vi "LvMPDC_SUB_SettingDialog.vi"(9 "Setting":T1) -> (1 "Setting out":T1, 2 "Caccel?":bool)   [LabVIEW 2012]
uses:
  LvMPDC_Typdef_Setting.ctl
  <vilib>/Utility/miscctls.llb/LVPointTypeDef.ctl
panel:
  in  "btn Test":bool
  in  "btn Cancel":bool
  in  "btn OK":bool
  in  "Port":u16=6600 caption="Port:"
  in  "server":string caption="Address:"
  # "MPD Server"
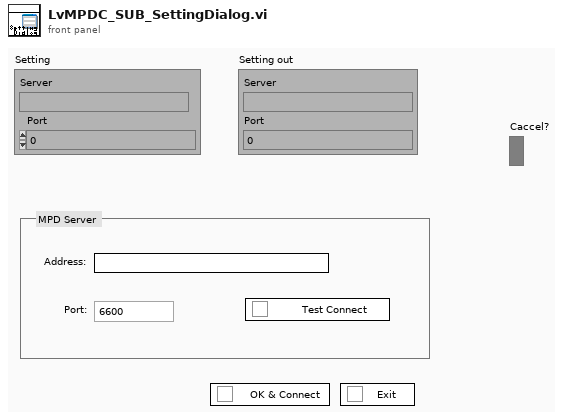
[diagram p1: front panel]
types:
  T1 = typedef "LvMPDC_Typdef_Setting.ctl" = cluster{"Server":string, "Port":u16}
  T2 = typedef "LVPointTypeDef.ctl" = cluster{"Horizontal":i16, "Vertical":i16}
  T3 = enum8{"Enabled", "Disabled", "Disabled and Grayed Out"}
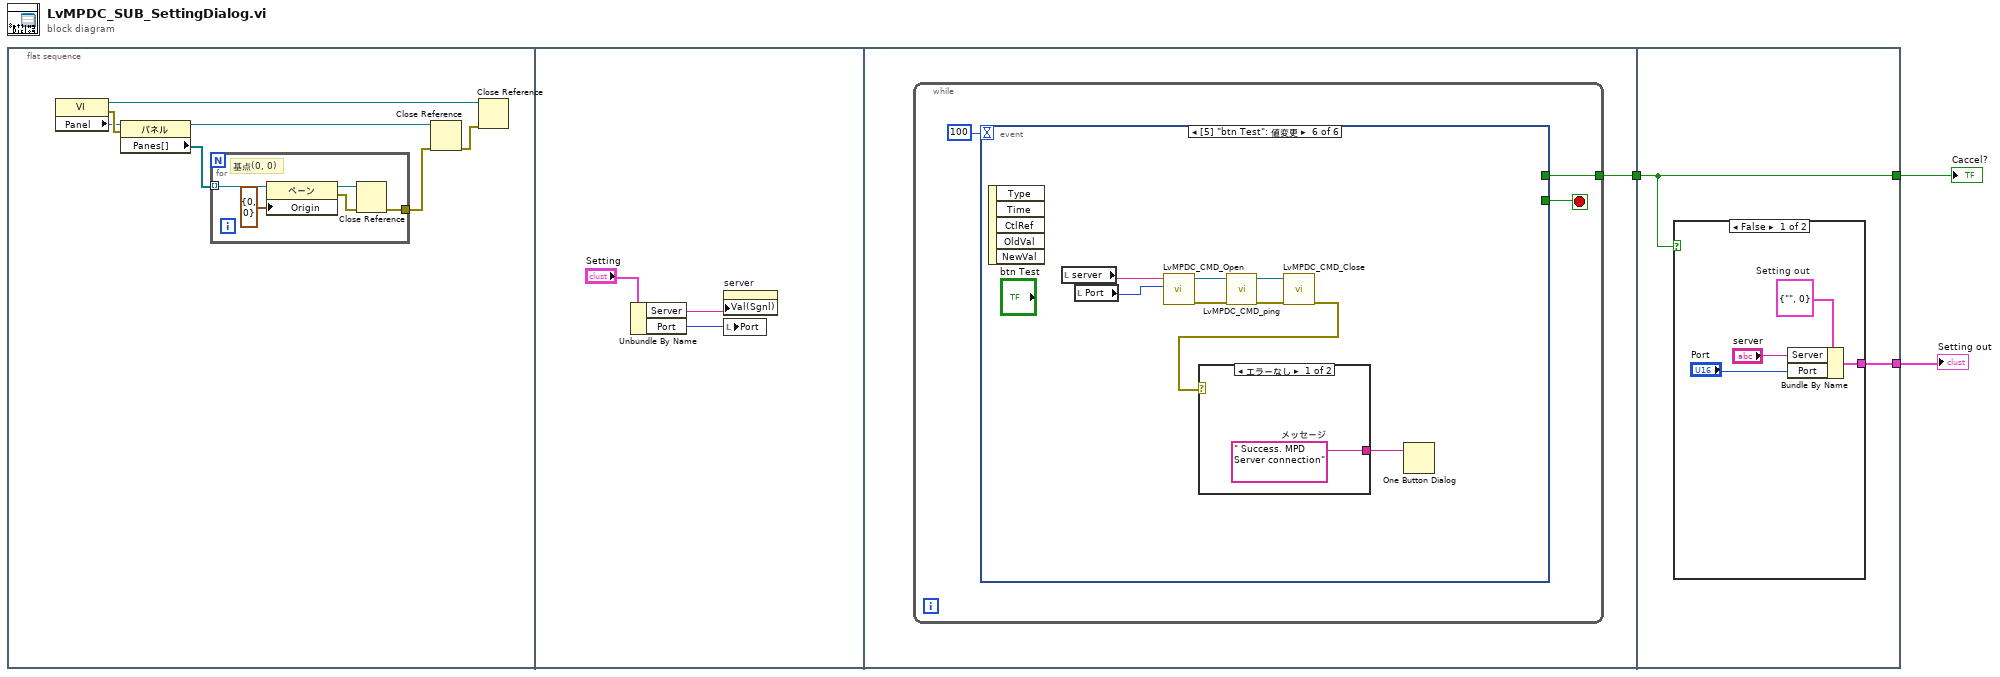
[diagram p0: block diagram]
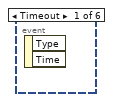
[diagram p2: hidden frame]
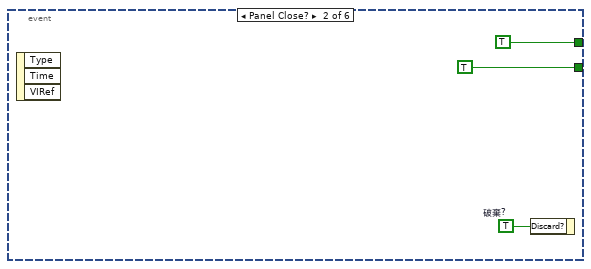
[diagram p3: hidden frame]
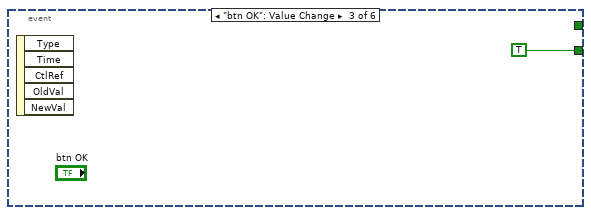
[diagram p4: hidden frame]
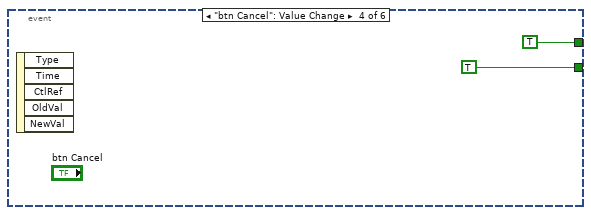
[diagram p5: hidden frame]
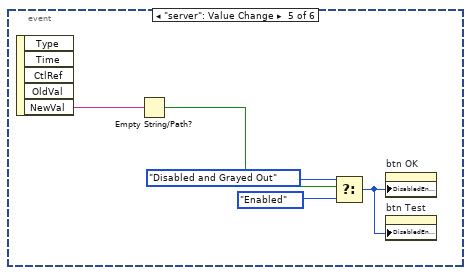
[diagram p6: hidden frame]
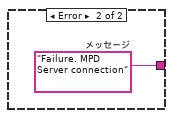
[diagram p7: hidden frame]
diagram:
  n1 = flat-sequence {
    tunnel: [w19] -> w3
    tunnel: w3 -> [w45]
    tunnel: [w45] -> w2
    tunnel: [w44] -> w1
    frame #0 {
      n2 = property class="VI"() -> (reference out=w7:refnum<vi>, error out=w10:errorcluster, "Panel"=w4:refnum<vi>)  [unwired: 2 in]
      n3 = property on="プロパティノード" class="パネル"(reference=w4, error in=w10) -> (reference out=w6:refnum<vi>, "Panes[]"=w5:refnum<vi>[])  [unwired: 1 out]
      n4 = for {
        tunnel: w5 -> [w15] mode=indexing
        tunnel: [w12] -> w8
        # "基点(0, 0)"
        n5 = property on="プロパティノード" class="ペーン"(reference=w15, "Origin"=T2 {"Horizontal"=0, "Vertical"=0} ("原点")) -> (reference out=w14:refnum<vi>, error out=w13:errorcluster)  [unwired: 1 in]
        n6 = Close Reference(reference=w14, error in (no error)=w13) -> (error out=w12:errorcluster)
      }
      n7 = Close Reference(reference=w6, error in (no error)=w8) -> (error out=w9:errorcluster)
      n8 = Close Reference(reference=w7, error in (no error)=w9) -> ()  [unwired: 1 out]
    }
    frame #1 {
      n9 = Unbundle By Name("Setting") -> ("Server"=w17:string, "Port"=w16:u16)
      n10 = property on="server" class="Str"("Val(Sgnl)"=w17) -> ()  [unwired: 2 in, 2 out]
      n11 = local write "Port"(w16) -> ()
    }
    frame #2 {
      n12 = while {
        tunnel: [w20] -> w19
        stop <- w21 stop-if-true
        n13 = event shown="[5] \"btn Test\": 値変更" {
          selector: _ -> [_ _ _ _ _ _]
          dyn-events: _ -> [_ _ _ _ _ _]
          timeout: 100 -> [_ _ _ _ _ _]
          tunnel: [_ TRUE TRUE TRUE _ _] -> w21
          tunnel: [_ TRUE _ TRUE _ _] -> w20
          event Timeout {
            n14 = event-data() -> ()  [unwired: 1 in, 2 out]
          }
          event Panel Close? {
            w25 = TRUE  # 破棄?
            n15 = event-data() -> ()  [unwired: 1 in, 3 out]
            n16 = event-data("Discard?"=w25) -> ()  [unwired: 1 in, 1 out]
          }
          event "btn OK": Value Change {
            n17 = event-data() -> ()  [unwired: 1 in, 5 out]
          }
          event "btn Cancel": Value Change {
            n18 = event-data() -> ()  [unwired: 1 in, 5 out]
          }
          event "server": Value Change {
            n19 = event-data() -> ("NewVal"=w33:string)  [unwired: 1 in, 4 out]
            n20 = Empty String/Path?(string/path=w33) -> (empty?=w32:bool)
            n21 = Select(t=T3."Disabled and Grayed Out", s=w32, f=T3."Enabled") -> (s? t:f=w29:T3)
            n22 = property on="btn OK" class="Bool"("DisabledEnum"=w29) -> ()  [unwired: 2 in, 2 out]
            n23 = property on="btn Test" class="Bool"("DisabledEnum"=w29) -> ()  [unwired: 2 in, 2 out]
          }
          event "btn Test": Value Change {
            n24 = event-data() -> ()  [unwired: 1 in, 5 out]
            n25 = local read "server"() -> (w37:string)
            n26 = local read "Port"() -> (w36:u16)
            n27 = call "LvMPDC_CMD_Open.vi"("Port"=w36, "Server"=w37) -> ("error out"=w40:errorcluster, "Connect ID out"=w41:refnum<k5>)  [unwired: 8 in]
            n28 = call "LvMPDC_CMD_ping.vi"("error in (no error)"=w40, "Connect ID"=w41) -> ("error out"=w38:errorcluster, "Connect ID out"=w39:refnum<k5>)  [unwired: 8 in]
            n29 = call "LvMPDC_CMD_Close.vi"("error in (no error)"=w38, "Connect ID"=w39) -> ("error out"=w35:errorcluster)  [unwired: 9 in]
            n30 = case shown="エラーなし" w35 {
              tunnel: [w42 w43] -> w34
              frame No Error {
                w42 = " Success. MPD Server connection"  # メッセージ
              }
              frame Error {
                w43 = "Failure. MPD Server connection"  # メッセージ
              }
            }
            n31 = One Button Dialog(message=w34) -> ()  [unwired: 1 in, 1 out]
          }
        }
      }
    }
    frame #3 {
      n32 = case shown="FALSE" w45 {
        tunnel: [w46 _] -> w44
        frame False {
          w49 = T1 {"Server"="", "Port"=0}  # Setting out
          n33 = Bundle By Name(cluster=w49, "Server"="server", "Port"="Port") -> (w46:T1)
        }
        frame True {
          # "Cancel"
        }
      }
    }
  }
  "Caccel?" <- w2
  "Setting out" <- w1
